vi "Model Check.vi"(8 "error in (no error)":errorcluster, 11 "VISA resource name":refnum<visa-resource-name>) -> (0 "error out":errorcluster, 1 "Model":u16(ring) items=["2601A", "2602A", "2611A", "2612A", "2635A", "2636A", "2657A", "2601B", "2602B", "2604B", "2606B", "2611B", "2612B", "2614B", "2634B", "2635B", "2636B", "2651A", "2604A", "2614A", "2634A"], 2 "Series":u16(ring) items=["2600A Series", "2600B Series"], 3 "VISA resource name out":refnum<visa-resource-name>)   [LabVIEW 2015, in "Keithley 2600 Series.lvlib"]
doc: "Indicates the instrument model type."
uses:
  Keithley 2600 Series.lvlib
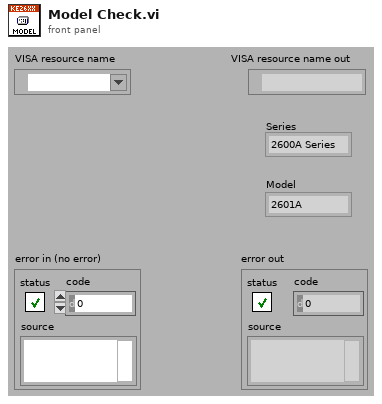
[diagram p1: front panel]
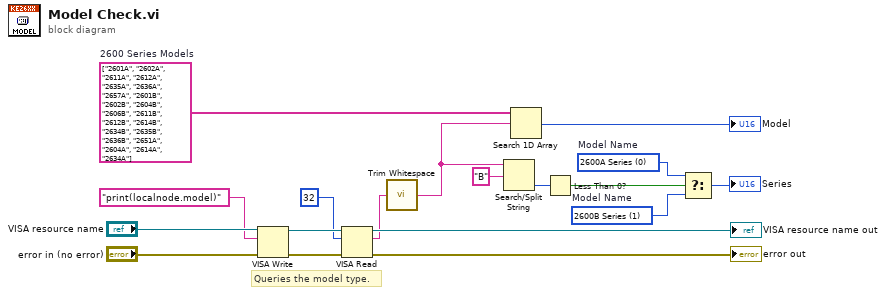
[diagram p0: block diagram]
diagram:
  w4 = u16 1 items=["2600A Series", "2600B Series"]  # Model Name
  w6 = u16 0 items=["2600A Series", "2600B Series"]  # Model Name
  w3 = string[] ["2601A", "2602A", "2611A", "2612A", "2635A", "2636A", "2657A", "2601B", "2602B", "2604B", "2606B", "2611B", "2612B", "2614B", "2634B", "2635B", "2636B", "2651A", "2604A", "2614A", "2634A"]  # 2600 Series Models
  # "Queries the model type."
  n1 = VISA Write(VISA resource name="VISA resource name", write buffer="print(localnode.model)", error in (no error)="error in (no error)") -> (VISA resource name out=w16:refnum<visa-resource-name>, error out=w15:errorcluster)  [unwired: 1 out]
  n2 = VISA Read(VISA resource name=w16, byte count=u32 32, error in (no error)=w15) -> (VISA resource name out=→"VISA resource name out":refnum<visa-resource-name>, read buffer=w10:string, error out=→"error out":errorcluster)  [unwired: 1 out]
  n3 = call <vilib>:"Trim Whitespace.vi"("string"=w10) -> ("trimmed string"=w1:string)  [unwired: 1 in]
  n4 = Search/Split String(string=w1, search string/char (-)="B") -> (offset of match=w8:i32)  [unwired: 1 in, 2 out]
  n5 = Search 1D Array(1D array=w3, element=w1) -> (index of element=→"Model":i32)  [unwired: 1 in]
  n6 = Less Than 0?(x=w8) -> (x < 0?=w7:bool)
  n7 = Select(t=w6, s=w7, f=w4) -> (s? t:f=→"Series":u16)
